vi "getChildrenArray.vi"(8 "error in (no error)":errorcluster, 11 "xmlNode.lvclass in":refnum<class "xmlNode.lvclass">) -> (0 "error out":errorcluster, 2 "Children":refnum<class "xmlNode.lvclass">[](array[class]), 3 "xmlNode.lvclass out":refnum<class "xmlNode.lvclass">)   [LabVIEW 2011, in "Tools.lvlib" / "xml.lvlib" / "xmlNode.lvclass"]
doc: "Gets all of the xml node children nodes.\ni.e. gets all the child xml elements of this example.\n\n<xml element>\n <child xml element 1> value </child xml element 1>\n <child xml element 2> value </child xml element 2>\n</xml element>"
uses:
  xmlNode.lvclass
  xmlNode.lvclass/xmlNode.ctl
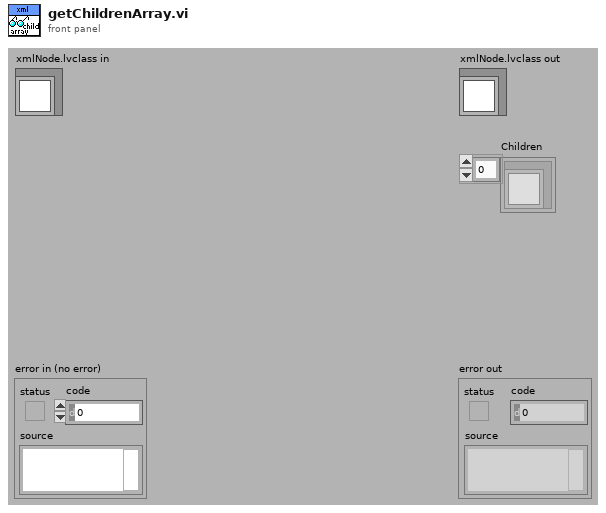
[diagram p1: front panel]
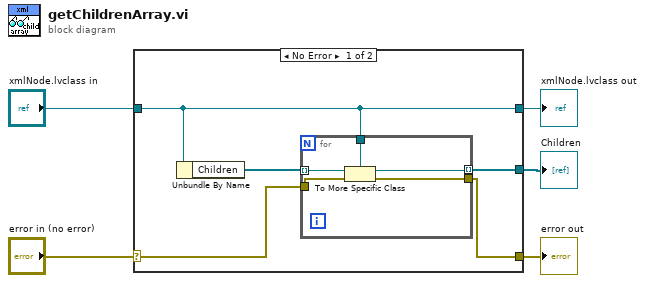
[diagram p0: block diagram]
diagram:
  n1 = case shown="No Error" "error in (no error)" {
    selector: "error in (no error)" -> [w9 w16]
    tunnel: [w8 w16] -> w4
    tunnel: [w6 w17] -> w2
    tunnel: "xmlNode.lvclass in" -> [w6 w17]
    tunnel: [w7 _] -> w1
    frame No Error {
      n2 = Unbundle By Name(w6) -> ("Children"=w10:refnum<class>[])
      n3 = for {
        tunnel: w10 -> [w15] mode=indexing
        tunnel: w9 -> [w14]
        tunnel: [w13] -> w8
        tunnel: [w12] -> w7 mode=indexing
        tunnel: w6 -> [w11]
        n4 = To More Specific Class(target class=w11, reference=w15, error in=w14) -> (specific class reference=w12:refnum<class "xmlNode.lvclass">, error out=w13:errorcluster)
      }
    }
    frame Error {
    }
  }
  "error out" <- w4
  "xmlNode.lvclass out" <- w2
  "Children" <- w1
